vi "SCP-Main.vi"() -> ()   [LabVIEW 2019]
doc: "The myRIO Project template acquires acceleration data from the onboard accelerometer and displays the changes of acceleration values in a waveform chart."
uses:
  <vilib>/myRIO/Instrument Drivers/Onboard IO/AI/typedefs/AI Reference.ctl
  <vilib>/myRIO/Common/Instrument Driver Framework/Utilities/typedefs/myRIO Generic Hardware Reference.ctl
  <vilib>/myRIO/Common/Instrument Driver Framework/Utilities/typedefs/Hardware Version Enum.ctl
  <vilib>/myRIO/Common/Instrument Driver Framework/Utilities/typedefs/myRIO v1.0 Reference.ctl
  <vilib>/myRIO/Common/Instrument Driver Framework/Utilities/typedefs/Generic FPGA Reference.ctl
  <vilib>/myRIO/Common/Instrument Driver Framework/myRIO v1.0/AI/typedefs/AI Channels List.ctl
  <vilib>/myRIO/Common/Instrument Driver Framework/myRIO v1.0/AI/typedefs/AI Channels Enum.ctl
  <vilib>/myRIO/Common/Instrument Driver Framework/Utilities/typedefs/Analog Scaling Constants List.ctl
  <vilib>/myRIO/Common/Instrument Driver Framework/Utilities/typedefs/Analog Scaling Constants.ctl
  <vilib>/userDefined/High Color/nirio_resource_hc.ctl
  <vilib>/myRIO/Common/Instrument Driver Framework/Utilities/vis/Is FPGA Ref Available.vi
  <vilib>/myRIO/Common/Instrument Driver Framework/myRIO v1.0/AI/vis/myRIO v1.1 Open AI.vi
  <vilib>/myRIO/Instrument Drivers/Onboard IO/AI/vis/Read.vi
  <vilib>/myRIO/Common/Instrument Driver Framework/Utilities/vis/Validate Channels.vi
  <vilib>/myRIO/Common/Instrument Driver Framework/myRIO v1.0/AI/vis/myRIO v1.0 Reserve AI.vi
  <vilib>/myRIO/Common/Instrument Driver Framework/myRIO v1.0/UART/vis/myRIO v1.0 Close UART.vi
  <vilib>/myRIO/Common/Instrument Driver Framework/myRIO v1.0/AI/vis/myRIO v1.0 Build MUX Configuration AI.vi
  <vilib>/myRIO/Common/Instrument Driver Framework/myRIO v1.0/Resource Manager/vis/myRIO v1.0 Reserve Channel List.vi
  <vilib>/myRIO/Common/Instrument Driver Framework/myRIO v1.0/Resource Manager/vis/myRIO v1.0 Reserve Channel.vi
  <vilib>/myRIO/Common/Instrument Driver Framework/myRIO v1.0/Resource Manager/vis/myRIO v1.0 Unreserve Channel.vi
  <vilib>/myRIO/Common/Instrument Driver Framework/myRIO v1.0/Resource Manager/vis/myRIO v1.0 Build Mutex Name.vi
  <vilib>/Utility/VariantDataType/GetNumericInfo.vi
  <vilib>/Utility/error.llb/Error Cluster From Error Code.vi
  <vilib>/myRIO/Common/Instrument Driver Framework/myRIO v1.0/myRIO v1.1 Open.vi
  <vilib>/myRIO/Common/Instrument Driver Framework/myRIO v1.0/AI/vis/myRIO v1.0 Get Scaling Constants AI.vi
  <vilib>/myRIO/Common/Instrument Driver Framework/Utilities/vis/IO Manager.vi
  <vilib>/myRIO/Common/Instrument Driver Framework/Utilities/vis/Configuration Manager.vi
  <vilib>/myRIO/Common/Instrument Driver Framework/myRIO v1.0/myRIO v1.0 Close.vi
  <vilib>/myRIO/Common/Instrument Driver Framework/myRIO v1.0/AI/vis/myRIO v1.0 Read AI.vi
  <vilib>/myRIO/Common/Instrument Driver Framework/Utilities/vis/FPGA Ref Manager.vi
  <vilib>/myRIO/Common/Instrument Driver Framework/myRIO v1.0/myRIO v1.0 Reset FPGA.vi
  <vilib>/myRIO/Common/Instrument Driver Framework/myRIO v1.0/IRQ/vis/myRIO v1.0 IRQ Info FGV.vi
  <vilib>/myRIO/Common/Instrument Driver Framework/myRIO v1.0/IRQ/vis/myRIO v1.0 Timer IRQ Info FGV.vi
  <vilib>/myRIO/Common/Instrument Driver Framework/myRIO v1.0/IRQ/vis/myRIO v1.0 ISR Agent.vi
  <vilib>/myRIO/Instrument Drivers/Utilities/vis/Reset Index.vi
  <vilib>/myRIO/Common/Instrument Driver Framework/myRIO v1.0/Resource Manager/vis/myRIO v1.0 Block Write Resource Manager.vi
  <vilib>/myRIO/Express VI/Onboard IO/AI/AI Express VI.xnode
  <vilib>/myRIO/Instrument Drivers/Onboard IO/AI/vis/myRIO AI Open.xnode
  <vilib>/myRIO/Instrument Drivers/Onboard IO/AI/AI.lvlib
  <vilib>/myRIO/Instrument Drivers/Utilities/Utilities.lvlib
panel:
  in  "Speed":dbl(slide) scale=0.0..1.0
  in  "Left":bool
  in  "Right":bool
  in  "Backward":bool
  in  "Forward":bool
  in  "RGBC\nSensor":bool
  in  "Distance\nSensor":bool
  in  "Reflection\nSensor":bool
  in  "Manual":bool
  out "Total B":u32
  out "Total R":u32
  out "Total G":u32
  out "RO7":dbl(slide) scale=0.0..5.0
  out "RO6":dbl(slide) scale=0.0..5.0
  out "RO5":dbl(slide) scale=0.0..5.0
  out "RO4":dbl(slide) scale=0.0..5.0
  out "RO3":dbl(slide) scale=0.0..5.0
  out "RO2":dbl(slide) scale=0.0..5.0
  out "RO1":dbl(slide) scale=0.0..5.0
  out "RO0":dbl(slide) scale=0.0..5.0
  out "DO0":dbl(knob) scale=0.0..5.0
  out "error out":errorcluster
  in  "Stop":bool
  # "Overview: SmartCityProject - This is the programmating for an automatic line-tracking robot.\nCurrent Features\n1. Gathering Data using sensors\n2. [WIP] Manual driving"
  # "DEBUG\nCONSOLE"
  # "ONLY MEANT FOR\nDEBUGGING, DO\nNOT TOUCH"
  # "DATA\nRS"
  # "DATA\nDS"
  # "ERROR\nLOG"
  # "(Connects to C/AI0)"
  # "DATA\nRGBS"
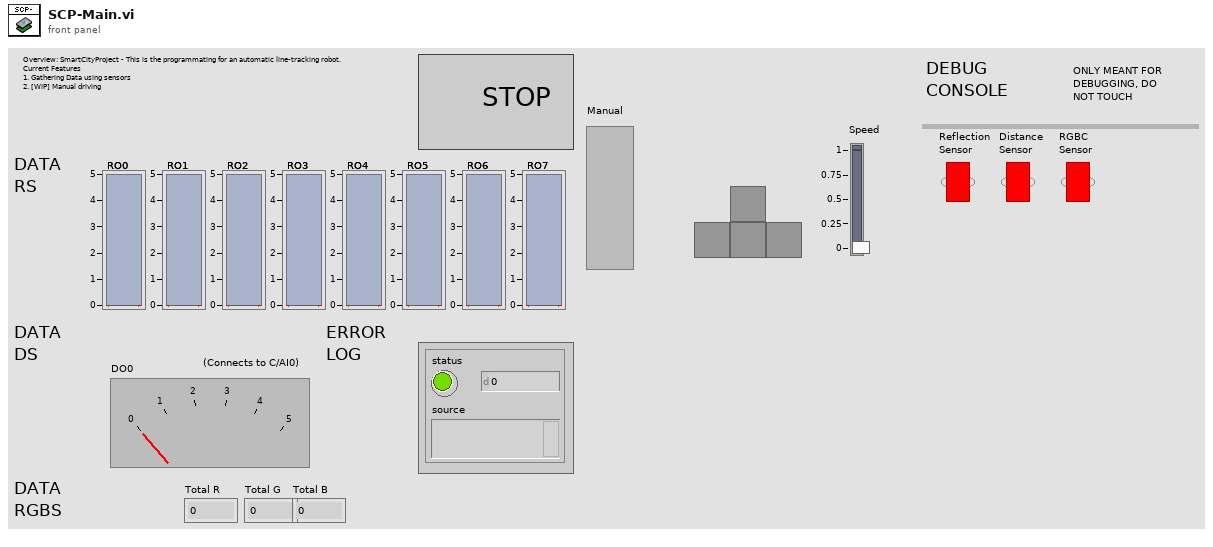
[diagram p1: front panel]
types:
  T1 = typedef "AI.lvlib/AI Reference.ctl" = cluster{"myRIO Reference":T2, "AI Channels List":T6, "AI Scaling Constants List":T8}
  T2 = typedef "myRIO Generic Hardware Reference.ctl" = cluster{"myRIO Model":T3, "myRIO Hardware Reference":T4}
  T3 = typedef "Hardware Version Enum.ctl" = enum16{"Unknown", "myRIO-1900", "myRIO-1950", "roboRIO", "NI ELVIS RIO CM", "ELVIS III"}
  T4 = typedef "myRIO v1.0 Reference.ctl" = cluster{"Generic FPGA Reference":T5, "Allow multiple opens":bool}
  T5 = typedef "Generic FPGA Reference.ctl" = refnum<k20>
  T6 = typedef "AI Channels List.ctl" = T7[]
  T7 = typedef "AI Channels Enum.ctl" = enum16{"Not Connected", "AudioIn/Left", "AudioIn/Right", "C/AI0", "C/AI1", "A/AI0", "A/AI1", "A/AI2", "A/AI3", "A/AI4", "A/AI5", "A/AI6", "A/AI7", "B/AI0", "B/AI1", "B/AI2", "B/AI3", "B/AI4", "B/AI5", "B/AI6", "B/AI7", "AI/AI0", "AI/AI1", "AI/AI2", "AI/AI3", "A/AI0 (DIFF)", "A/AI1 (DIFF)", "A/AI2 (DIFF)", "A/AI3 (DIFF)", "B/AI0 (DIFF)", "B/AI1 (DIFF)", "B/AI2 (DIFF)", "B/AI3 (DIFF)"}
  T8 = typedef "Analog Scaling Constants List.ctl" = T9[]
  T9 = typedef "Analog Scaling Constants.ctl" = cluster{"LSB Weight (Volts)":dbl, "Offset (Volts)":dbl, "Signed?":bool}
  T10 = typedef "nirio_resource_hc.ctl" = tag
  T11 = cluster{"Values[0]":dbl, "Values[1]":dbl, "Values[2]":dbl, "Values[3]":dbl, "Values[4]":dbl, "Values[5]":dbl, "Values[6]":dbl, "Values[7]":dbl, "Values[8]":dbl}
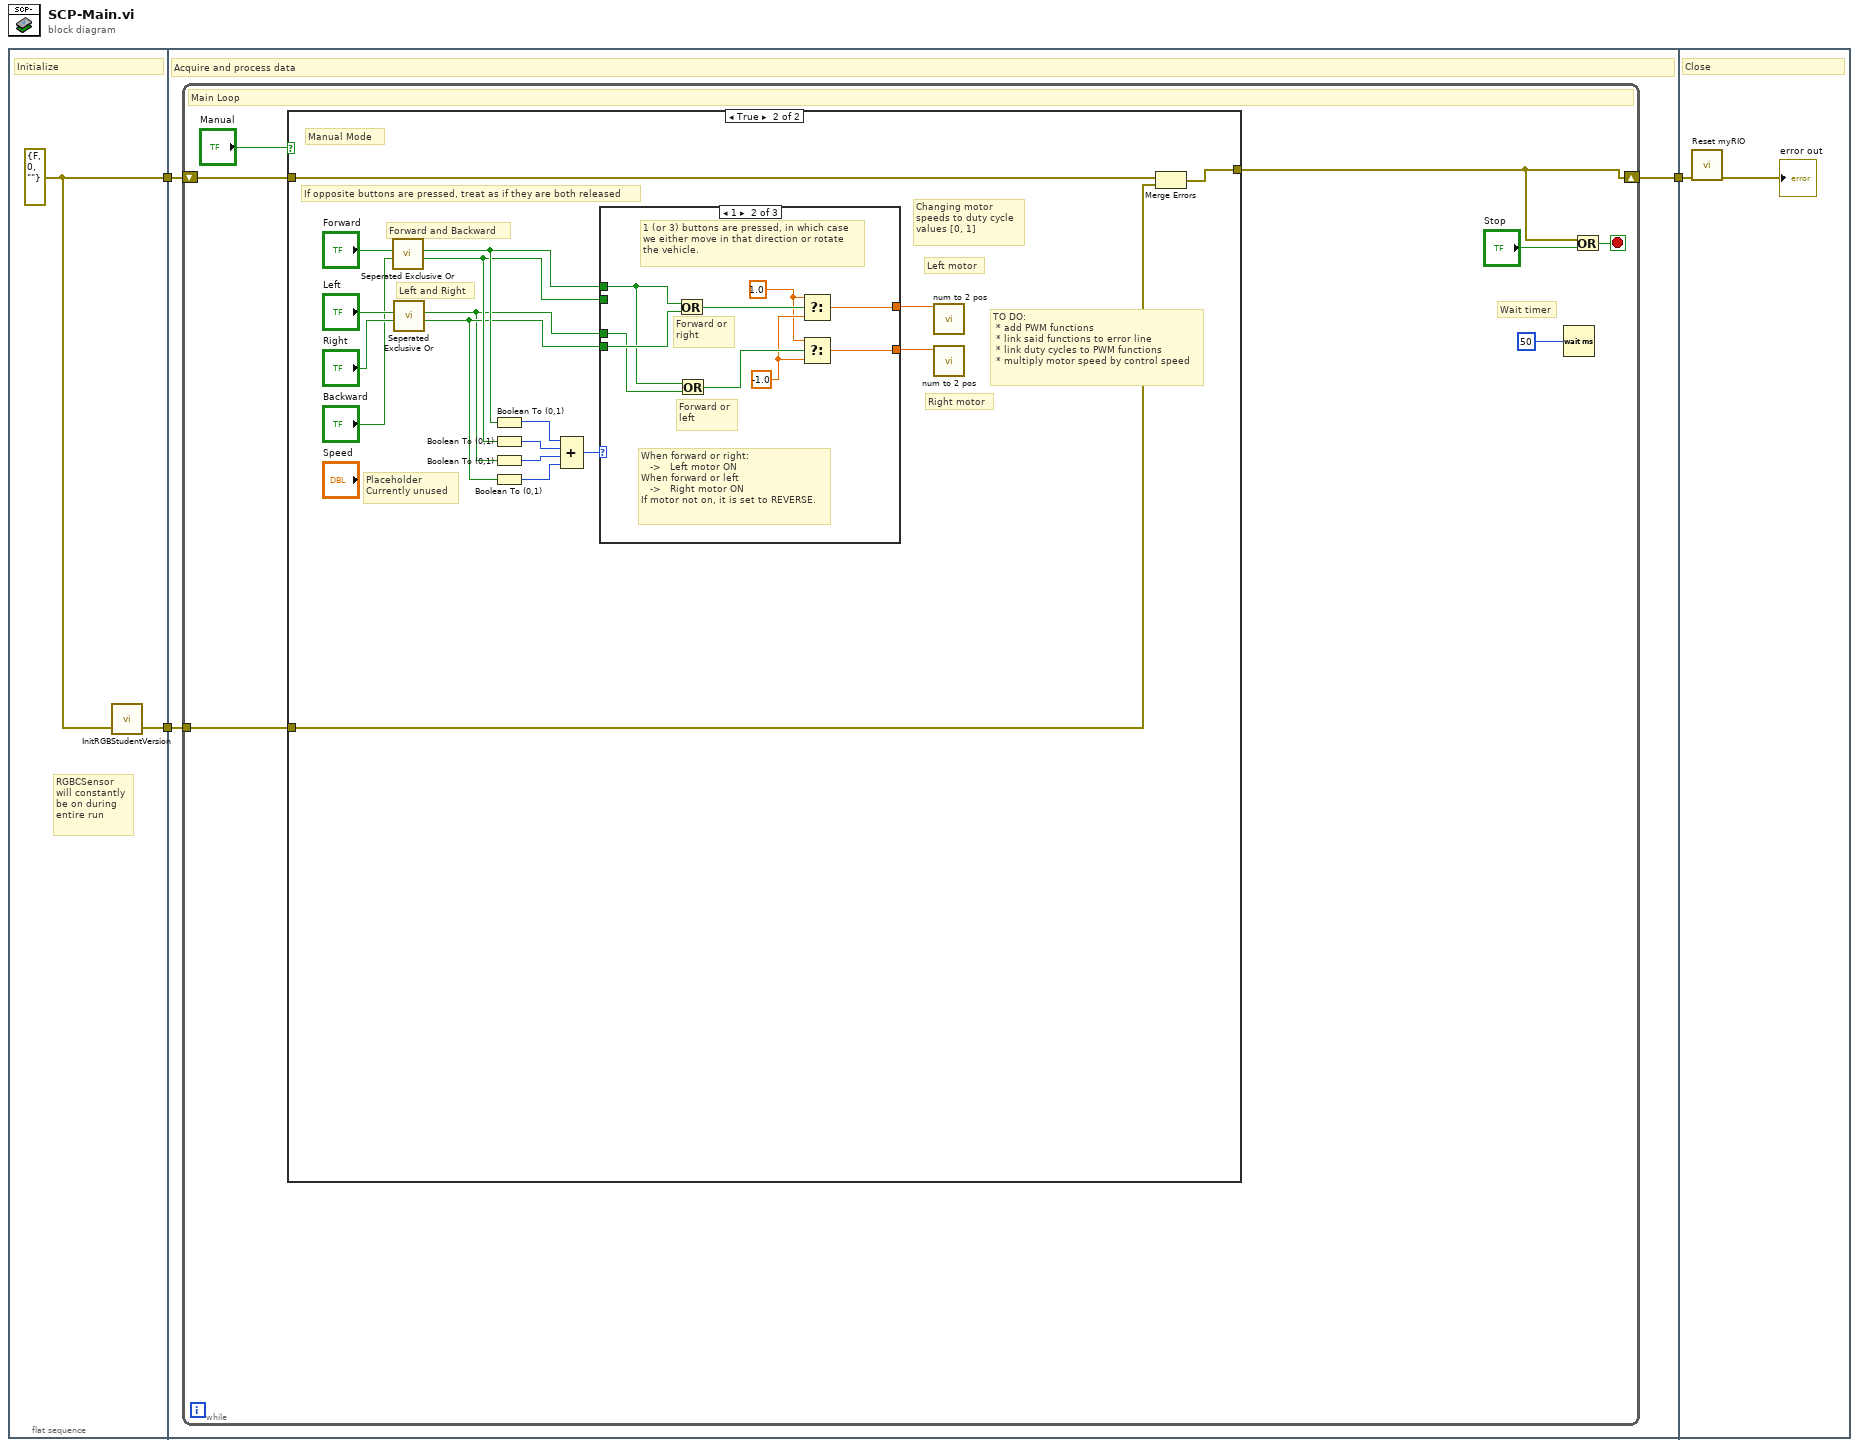
[diagram p0: block diagram]
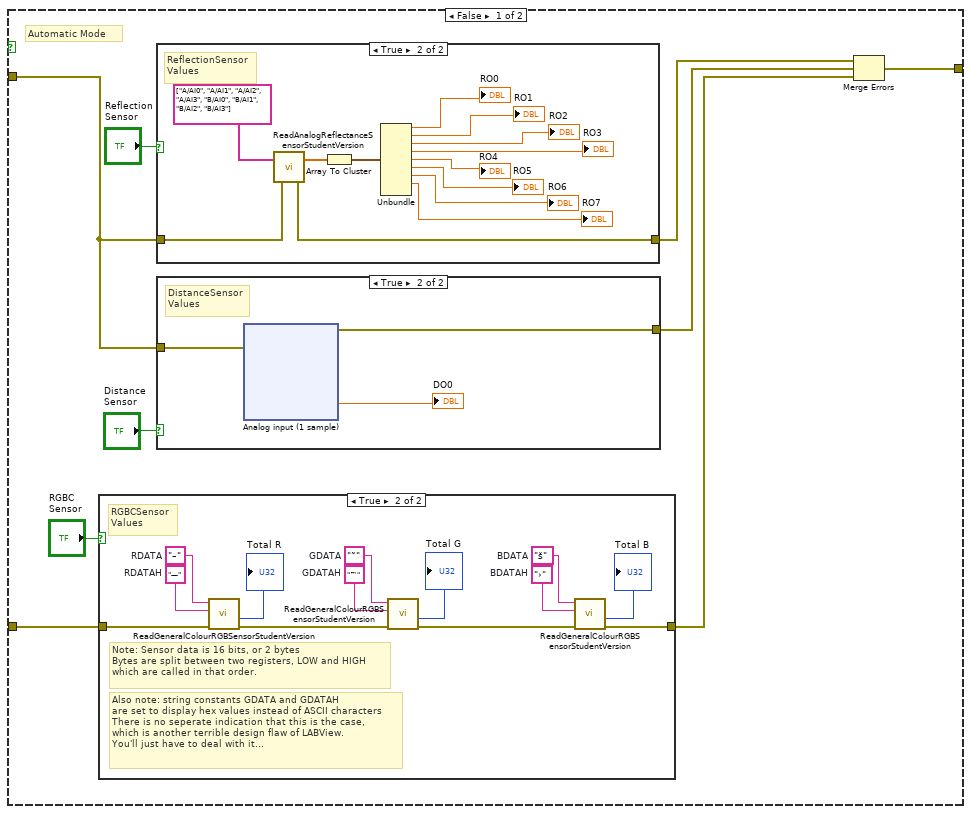
[diagram p2: hidden frame]
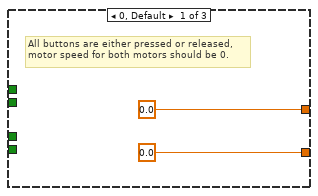
[diagram p6: hidden frame]
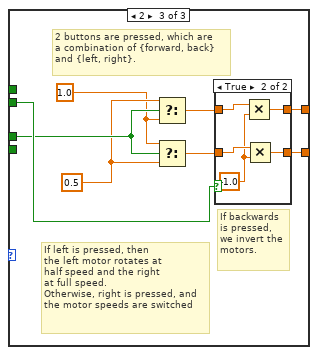
[diagram p7: hidden frame]
diagram:
  n1 = flat-sequence {
    tunnel: [w5] -> w3
    tunnel: [w4] -> w2
    tunnel: w3 -> [w8]
    tunnel: [w7] -> w1
    tunnel: w2 -> [w6]
    tunnel: w1 -> [w139]
    frame #0 {
      w5 = errorcluster {"status"=FALSE, "code"=0, "source"=""} ("error in (no error)")
      # "RGBCSensor\nwill constantly\nbe on during\nentire run"
      # "Initialize"
      n2 = call "InitRGBStudentVersion.vi"("error in (no error)"=w5) -> ("error out"=w4:errorcluster)  [unwired: 2 in]
    }
    frame #1 {
      # "Acquire and process data"
      n3 = while {
        shift-right: [w9] -> w7
        shift-left: w8 -> [w13]
        tunnel: w6 -> [w12]
        stop <- w15 stop-if-true
        # "Wait timer"
        # "Main Loop"
        n4 = case shown="True" "Manual" {
          tunnel: w13 -> [w23 w111]
          tunnel: w12 -> [w22 w109]
          tunnel: [w16 w110] -> w9
          frame False {
            # "Automatic Mode"
            n5 = case shown="True" "RGBC\nSensor" {
              tunnel: w22 -> [w25 w32]
              tunnel: [w25 w29] -> w17
              frame False {
              }
              frame True {
                w33 = "›"  # BDATAH
                w34 = "š"  # BDATA
                w35 = "—"  # RDATAH
                w36 = "–"  # RDATA
                w37 = "™"  # GDATAH
                w38 = "˜"  # GDATA
                # "RGBCSensor\nValues"
                # "Also note: string constants GDATA and GDATAH\nare set to display hex values instead of ASCII characters\nThere is no seperate indication that this is the case,\nwhich is another terrible design flaw of LABView.\nYou'll just have to deal with it..."
                # "Note: Sensor data is 16 bits, or 2 bytes\nBytes are split between two registers, LOW and HIGH\nwhich are called in that order."
                n6 = call "ReadGeneralColourRGBSensorStudentVersion.vi"("error in (no error)"=w32, "High"=w35, "Low"=w36) -> ("error out"=w31:errorcluster, "Total"=→"Total R":u32)  [unwired: 5 in, 2 out]
                n7 = call "ReadGeneralColourRGBSensorStudentVersion.vi"("error in (no error)"=w31, "High"=w37, "Low"=w38) -> ("error out"=w30:errorcluster, "Total"=→"Total G":u32)  [unwired: 5 in, 2 out]
                n8 = call "ReadGeneralColourRGBSensorStudentVersion.vi"("error in (no error)"=w30, "High"=w33, "Low"=w34) -> ("error out"=w29:errorcluster, "Total"=→"Total B":u32)  [unwired: 5 in, 2 out]
              }
            }
            n9 = case shown="True" "Reflection\nSensor" {
              tunnel: [w80 w93] -> w24
              tunnel: w23 -> [w80 w92]
              frame False {
              }
              frame True {
                # "ReflectionSensor\nValues"
                n10 = call "ReadAnalogReflectanceSensorStudentVersion.vi"("error in (no error)"=w92, "Channel Names"=tag[] ["A/AI0", "A/AI1", "A/AI2", "A/AI3", "B/AI0", "B/AI1", "B/AI2", "B/AI3"]) -> ("error out"=w93:errorcluster, "Values"=w90:dbl[])
                n11 = Array To Cluster(array=w90) -> (cluster=w89:T11)
                n12 = Unbundle(w89) -> ("Values[0]"=→"RO0":dbl, "Values[1]"=→"RO1":dbl, "Values[2]"=→"RO2":dbl, "Values[3]"=→"RO3":dbl, "Values[4]"=→"RO4":dbl, "Values[5]"=→"RO5":dbl, "Values[6]"=→"RO6":dbl, "Values[7]"=→"RO7":dbl)  [unwired: 1 out]
              }
            }
            n13 = case shown="True" "Distance\nSensor" {
              tunnel: w23 -> [w39 w42]
              tunnel: [w39 w41] -> w18
              frame False {
              }
              frame True {
                # "DistanceSensor\nValues"
                n14 = xnode "Analog input (1 sample)"("error in (no error)"=w42) -> ("C/AI0 (AI0)"=→"DO0":dbl, "error out"=w41:errorcluster)
              }
            }
            n15 = Merge Errors(w24, w18, w17) -> (w16:errorcluster)
          }
          frame True {
            # "Placeholder\nCurrently unused"
            # "Manual Mode"
            # "TO DO:\n * add PWM functions\n * link said functions to error line\n * link duty cycles to PWM functions\n * multiply motor speed by control speed"
            # "If opposite buttons are pressed, treat as if they are both released"
            # "Changing motor\nspeeds to duty cycle\nvalues [0, 1]"
            # "Right motor"
            # "Left motor"
            # "Left and Right"
            # "Forward and Backward"
            n16 = call "Seperated Exclusive Or.vi"("q"="Backward", "p"="Forward") -> ("only q"=w96:bool, "only p"=w97:bool)  [unwired: 8 in]
            n17 = call "Seperated Exclusive Or.vi"("q"="Right", "p"="Left") -> ("only q"=w95:bool, "only p"=w94:bool)  [unwired: 8 in]
            n18 = Boolean To (0,1)(Boolean=w97) -> (0, 1=w104:i16)
            n19 = Boolean To (0,1)(Boolean=w96) -> (0, 1=w103:i16)
            n20 = Boolean To (0,1)(Boolean=w94) -> (0, 1=w102:i16)
            n21 = Boolean To (0,1)(Boolean=w95) -> (0, 1=w101:i16)
            n22 = Compound Arithmetic op=ADD(w104, w103, w102, w101) -> (w100:i16)
            n23 = case shown="1" w100 {
              tunnel: [0.0 w121 w126] -> w99
              tunnel: [0.0 w122 w128] -> w98
              tunnel: w97 -> [_ w115 _]
              tunnel: w96 -> [_ _ w130]
              tunnel: w95 -> [_ w118 _]
              tunnel: w94 -> [_ w114 w125]
              frame 0, Default {
                # "All buttons are either pressed or released, \nmotor speed for both motors should be 0."
              }
              frame 1 {
                w117 = -1.0
                w116 = 1.0
                # "When forward or right:\n   ->   Left motor ON\nWhen forward or left\n   ->   Right motor ON\nIf motor not on, it is set to REVERSE."
                # "Forward or\nleft"
                # "Forward or\nright"
                # "1 (or 3) buttons are pressed, in which case\nwe either move in that direction or rotate\nthe vehicle."
                n24 = Or(x=w115, y=w118) -> (x .or. y?=w120:bool)
                n25 = Or(x=w115, y=w114) -> (x .or. y?=w119:bool)
                n26 = Select(t=w116, s=w120, f=w117) -> (s? t:f=w122:dbl)
                n27 = Select(t=w116, s=w119, f=w117) -> (s? t:f=w121:dbl)
              }
              frame 2 {
                w124 = 0.5
                w123 = 1.0
                # "If left is pressed, then\nthe left motor rotates at\nhalf speed and the right\nat full speed.\nOtherwise, right is pressed, and\nthe motor speeds are switched"
                # "If backwards\nis pressed,\nwe invert the\nmotors."
                # "2 buttons are pressed, which are\na combination of {forward, back}\nand {left, right}."
                n28 = Select(t=w124, s=w125, f=w123) -> (s? t:f=w129:dbl)
                n29 = Select(t=w123, s=w125, f=w124) -> (s? t:f=w127:dbl)
                n30 = case shown="True" w130 {
                  tunnel: w129 -> [w132 w137]
                  tunnel: [w132 w136] -> w128
                  tunnel: w127 -> [w131 w135]
                  tunnel: [w131 w133] -> w126
                  frame False {
                  }
                  frame True {
                    w134 = -1.0
                    n31 = Multiply(x=w137, y=w134) -> (x*y=w136:dbl)
                    n32 = Multiply(x=w135, y=w134) -> (x*y=w133:dbl)
                  }
                }
              }
            }
            n33 = call "num to 2 pos.vi"("Motorspeed"=w98) -> ()  [unwired: 9 in, 2 out]
            n34 = call "num to 2 pos.vi"("Motorspeed"=w99) -> ()  [unwired: 9 in, 2 out]
            n35 = Merge Errors(w111, w109) -> (w110:errorcluster)
          }
        }
        n36 = Wait (ms)(milliseconds to wait=50) -> ()  [unwired: 1 out]
        n37 = Or(x=w9, y="Stop") -> (x .or. y?=w15:bool)
      }
    }
    frame #2 {
      # "Close"
      n38 = call <vilib>:"Reset myRIO.vi"("error in (no error)"=w139) -> ("error out"=→"error out":errorcluster)  [unwired: 10 in]
    }
  }
